vi "Read Element of Product Installers Definition.vi"(8 "error in (no error)":errorcluster, 10 "Selected Product File Name":string, 11 "Bundle Builder in":refnum<class "Bundle Builder.lvclass">) -> (0 "error out":errorcluster, 2 "Product Installer":T1 caption="NI Product Installer / Custom Product Installer", 3 "Bundle Builder out":refnum<class "Bundle Builder.lvclass">)   [LabVIEW 2020, in "Bundle Builder.lvclass"]
uses:
  Bundle Builder.lvclass
  Typedef/Product Installer Definition.ctl
  Bundle Builder.lvclass/Bundle Builder.ctl
  92f76918-1563-4c6f-99b4-6a0cba476cd6.vi
  <vilib>/Comparison/Equal/Equal Functor/Equal Functor.lvclass
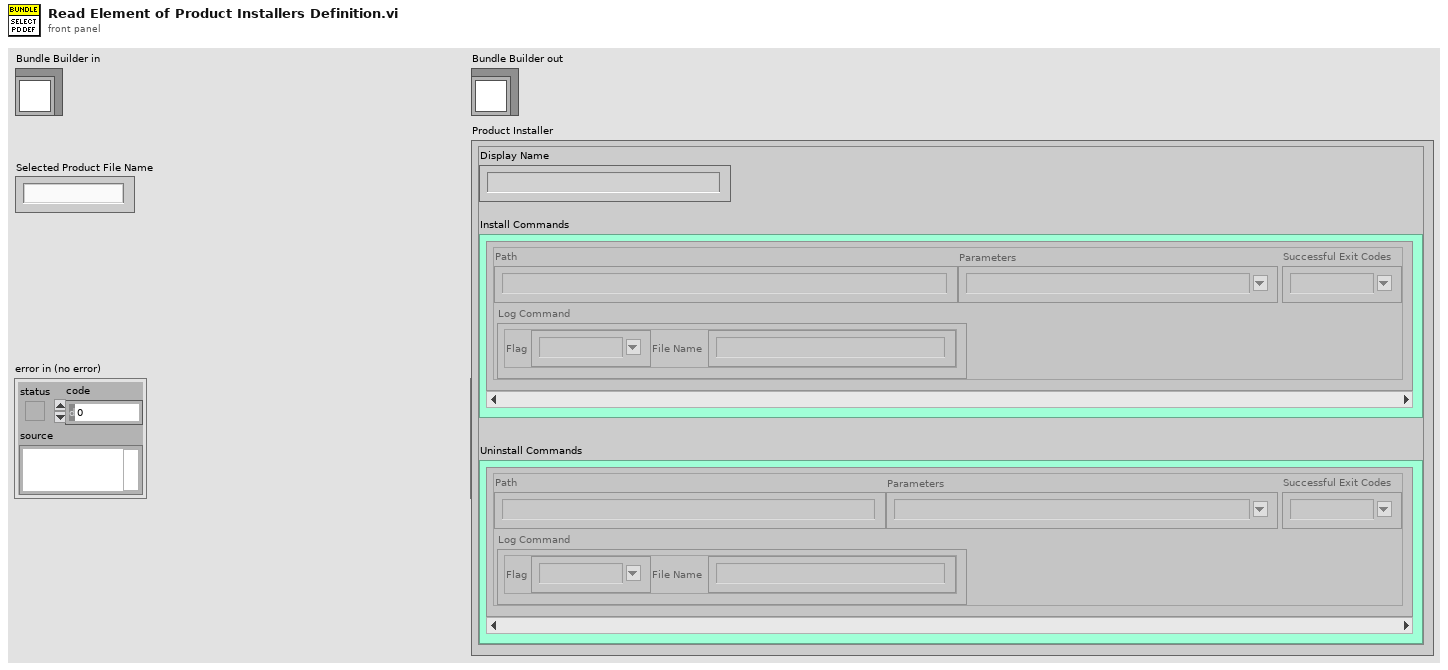
[diagram p1: front panel]
types:
  T1 = typedef "Product Installer Definition.ctl" = cluster{"Display Name":string, "Install Commands":cluster{"Path":string, "Parameters":string, "Successful Exit Codes":string, "Log Command":cluster{"Flag":string, "File Name":string}}[], "Uninstall Commands":cluster{"Path":string, "Parameters":string, "Successful Exit Codes":string, "Log Command":cluster{"Flag":string, "File Name":string}}[]}
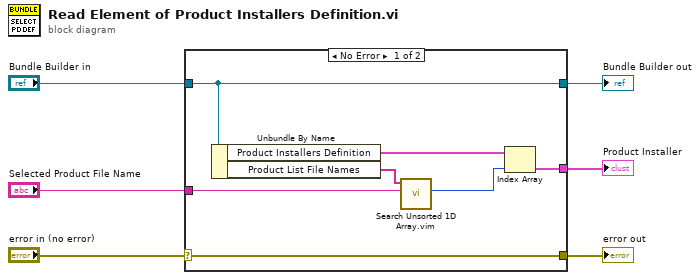
[diagram p0: block diagram]
diagram:
  n1 = case shown="No Error" "error in (no error)" {
    selector: "error in (no error)" -> [w13 w14]
    tunnel: [w13 w14] -> w5
    tunnel: [w12 w15] -> w3
    tunnel: "Bundle Builder in" -> [w12 w15]
    tunnel: [w10 _] -> w2
    tunnel: "Selected Product File Name" -> [w8 _]
    frame No Error {
      n2 = Unbundle By Name(w12) -> ("Product Installers Definition"=w11:T1[], "Product List File Names"=w9:string[])
      n3 = call "Search Unsorted 1D Array.vim"("element"=w8, "unsorted 1D array"=w9) -> ("index of element"=w7:i32)  [unwired: 9 in]
      n4 = Index Array(array=w11, index=w7) -> (element=w10:T1)
    }
    frame Error {
    }
  }
  "error out" <- w5
  "Bundle Builder out" <- w3
  "Product Installer" <- w2
